vi "Init Config.vi"(8 "error in":errorcluster) -> (0 "error out":errorcluster, 3 "Configuration":T1)   [LabVIEW 2020, in "CML UI.lvlib" / "Configuration.lvclass"]
doc: "Initialize the configuration for this module.\n____\nPeloton Config 2.0.0.9\nCopyright (c) 2024, Peloton"
uses:
  Configuration.lvclass
  Configuration--cluster.ctl
  C:/Program Files (x86)/National Instruments/LabVIEW 2020/vi.lib/Peloton/Peloton Config/DCFG Framework/Configuration_class/Configuration.lvclass
  <vilib>/Peloton/Peloton Config/DCFG Framework/Configuration_class/Configuration.lvclass/Configuration.ctl
  Configuration.lvclass/Configuration.ctl
  <vilib>/Peloton/Peloton Config/DCFG Framework/Configuration_class/Set Name.vi
  <vilib>/Peloton/Peloton Config/DCFG Framework/Configuration_class/Set File.vi
  <vilib>/Peloton/Peloton Config/DCFG Framework/Configuration_class/Set Order.vi
  <vilib>/Peloton/Peloton Config/DCFG Framework/Configuration_class/Set UIs.vi
  <vilib>/Peloton/Peloton Config/DCFG Framework/Configuration_class/Set Views.vi
  Set Configuration.vi
  UI - main UI setting.vi
  <vilib>/Peloton/Peloton Config/DCFG Framework/Peloton_lib_DCFG Framework.lvlib
  <vilib>/Peloton/Peloton Config/DCFG Framework/Configuration_class/Configuration.lvclass
  CML UI.lvlib
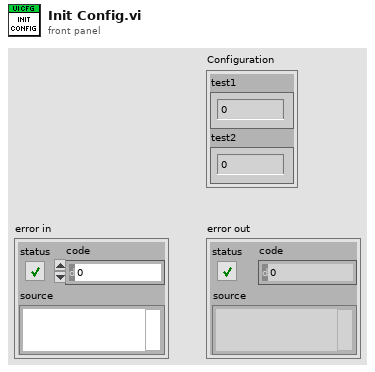
[diagram p1: front panel]
types:
  T1 = typedef "CML UI.lvlib/Configuration.lvclass/Configuration--cluster.ctl" = cluster{"test1":dbl, "test2":dbl}
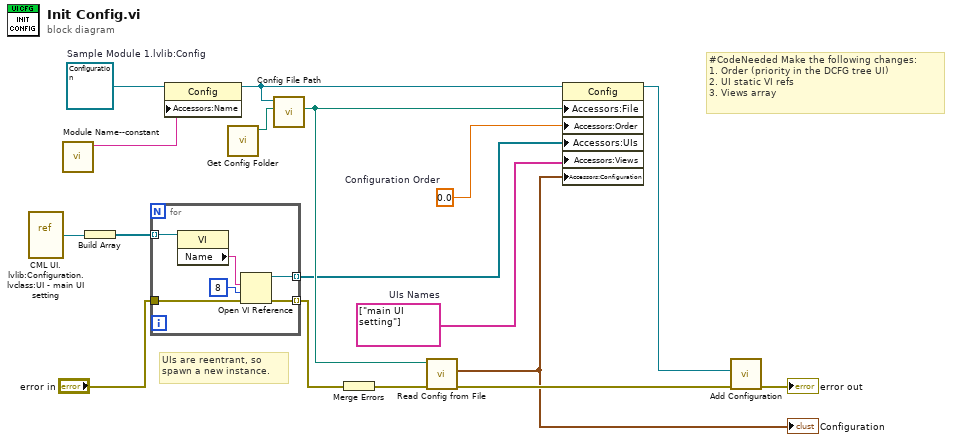
[diagram p0: block diagram]
diagram:
  w14 = string[] ["main UI setting"]  # UIs Names
  w16 = 0.0  # Configuration Order
  w13 = refnum<class "Configuration.lvclass"> refnum  # Sample Module 1.lvlib:Config
  # "UIs are reentrant, so spawn a new instance."
  # "#CodeNeeded Make the following changes:\n1. Order (priority in the DCFG tree UI)\n2. UI static VI refs\n3. Views array"
  n1 = vi-ref "CML UI.lvlib:Configuration.lvclass:UI - main UI setting.vi"() -> (w1:refnum<vi>)
  n2 = call "Module Name--constant.vi"() -> ("Module Name"=w8:string)  [unwired: 11 in]
  n3 = Build Array "Build Array"(w1) -> (w6:refnum<vi>[])
  n4 = for {
    tunnel: [w21] -> w3 mode=indexing
    tunnel: w6 -> [w18] mode=indexing
    tunnel: "error in" -> [w23]
    tunnel: [w22] -> w4 mode=indexing
    n5 = property class="VI"(reference=w18) -> ("Name"=w19:string)  [unwired: 1 in, 2 out]
    n6 = Open VI Reference(vi path=w19, options=8, error in (no error)=w23) -> (vi reference=w21:refnum<vi>, error out=w22:errorcluster)  [unwired: 3 in]
  }
  n7 = property class="Config"(reference=w13, "Accessors:Name"=w8) -> (reference out=w9:refnum<class "Configuration.lvclass">)  [unwired: 1 in, 1 out]
  n8 = call <vilib>:"Get Config Folder.vi"() -> ("Config Folder"=w2:path)  [unwired: 9 in, 2 out]
  n9 = call <vilib>:"Config File Path.vi"("Config Folder"=w2, "Config"=w9) -> ("Config File Path"=w15:path)  [unwired: 9 in]
  n10 = Merge Errors(w4) -> (w7:errorcluster)
  n11 = call "Read Config from File.vi"("error in"=w7, "Config File"=w15) -> ("error out"=w11:errorcluster, "Configuration"=w10:T1)  [unwired: 8 in]
  "Configuration" <- w10
  n12 = property class="Config"(reference=w9, "Accessors:File"=w15, "Accessors:Order"=w16, "Accessors:UIs"=w3, "Accessors:Views"=w14, "Accessors:Configuration"=w10) -> (reference out=w12:refnum<class "Configuration.lvclass">)  [unwired: 1 in, 1 out]
  n13 = call <vilib>:"Add Configuration.vi"("error in"=w11, "Config"=w12) -> ("error out"=→"error out":errorcluster)  [unwired: 9 in]
